vi "Ping return.vi"(8 "error in (no error)":errorcluster, 9 "Reception":T1, 10 "Emission":T1, 11 "UI_Actor in":refnum<class "UI_Actor.lvclass">) -> (0 "error out":errorcluster, 3 "UI_Actor out":refnum<class "UI_Actor.lvclass">)   [LabVIEW 2020, in "UI_Actor.lvlib" / "UI_Actor.lvclass"]
uses:
  UI_Actor.lvclass
  D:/Projets/STEP AT/UI Actor/support/Actor Framework.lvlibp/1abvi3w/vi.lib/ActorFramework/Actor/Actor.lvclass
  ctl_Ping payload.ctl
  UI_Actor.lvclass/UI_Actor.ctl
  UI_Actor Messages/Ping return Msg/Ping return Msg.lvclass/Ping return Msg.ctl
  support/Actor Framework.lvlibp/1abvi3w/vi.lib/ActorFramework/Message Enqueuer/Enqueue.vi
  UI_Actor Messages/Ping return Msg/Ping return Msg.lvclass
  support/Actor Framework.lvlibp/1abvi3w/vi.lib/ActorFramework/Actor/Actor.lvclass
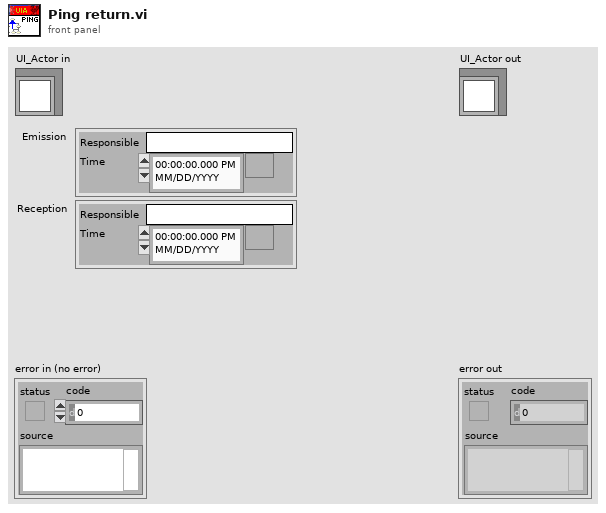
[diagram p1: front panel]
types:
  T1 = typedef "UI_Actor.lvlib/UI_Actor.lvclass/ctl_Ping payload.ctl" = cluster{"Responsible":string, "Time":timestamp}
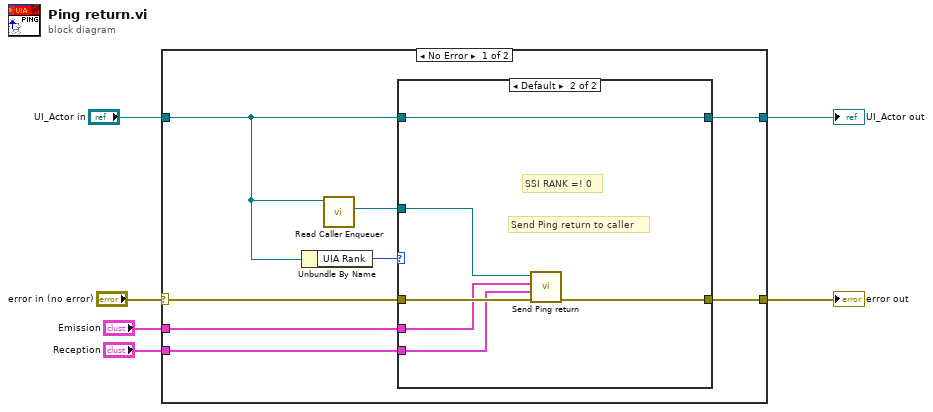
[diagram p0: block diagram]
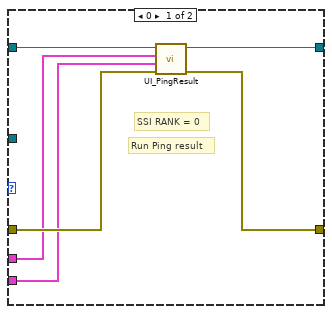
[diagram p2: hidden frame]
diagram:
  n1 = case shown="No Error" "error in (no error)" {
    selector: "error in (no error)" -> [w12 w28]
    tunnel: [w11 w28] -> w5
    tunnel: [w7 w27] -> w3
    tunnel: "UI_Actor in" -> [w8 w27]
    tunnel: "Emission" -> [w10 _]
    tunnel: "Reception" -> [w9 _]
    frame No Error {
      n2 = Unbundle By Name(w8) -> ("UIA Rank"=w14:i32)
      n3 = call "Read Caller Enqueuer.vi"("Actor"=w8) -> ("Caller Enqueuer"=w13:refnum<class "Message Enqueuer.lvclass">)  [unwired: 10 in]
      n4 = case shown="Default" w14 {
        tunnel: w12 -> [w18 w24]
        tunnel: [w17 w25] -> w11
        tunnel: w13 -> [_ w26]
        tunnel: w10 -> [w16 w23]
        tunnel: w9 -> [w15 w22]
        tunnel: w8 -> [w20 w21]
        tunnel: [w19 w21] -> w7
        frame 0 {
          # "SSI RANK = 0"
          # "Run Ping result"
          n5 = call-dynamic "UI_PingResult.vi"("error in (no error)"=w18, "Reception"=w15, "Emission"=w16, "UI_Actor in"=w20) -> ("error out"=w17:errorcluster, "UI_Actor out"=w19:refnum<class "UI_Actor.lvclass">)  [unwired: 6 in]
        }
        frame Default {
          # "Send Ping return to caller"
          # "SSI RANK =! 0"
          n6 = call "Send Ping return.vi"("error in (no error)"=w24, "Reception"=w22, "Emission"=w23, "Message Enqueuer"=w26) -> ("error out"=w25:errorcluster)  [unwired: 6 in, 1 out]
        }
      }
    }
    frame Error {
    }
  }
  "error out" <- w5
  "UI_Actor out" <- w3
